vi "Wait on Response.vi"(8 "error in":errorcluster {"code" format="Error %.0f"}, 10 "timeout in ms (-1)":i32=-1, 11 "NATS Subscriber in":refnum<class "NATS Subscription.lvclass">) -> (0 "error out":errorcluster {"code" format="Error %.0f"}, 2 "time out":bool, 3 "nats message":T1)   [LabVIEW 2020, in "NATS Subscription.lvlib" / "NATS Subscription.lvclass"]
doc: "Returns the next subscription response."
uses:
  NATS Subscription.lvclass
  NATS Subscription.lvclass/NATS Subscription.ctl
  <vilib>/NATS/NATS Core/Controls/msg type.ctl
  <vilib>/NATS/NATS Core/NATS Core.lvlib
  <vilib>/NATS/NATS Core/Controls/nats message.ctl
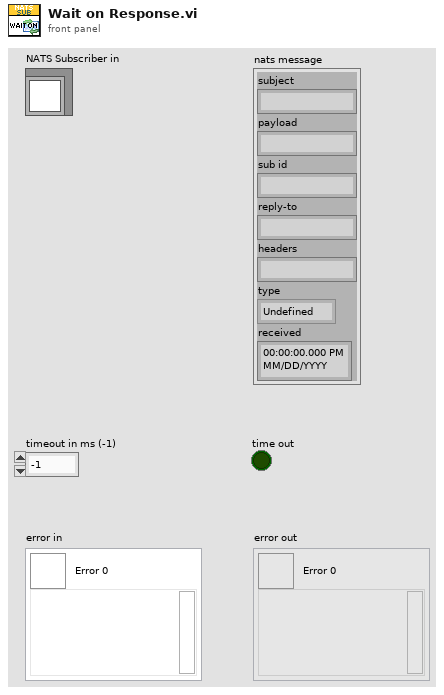
[diagram p1: front panel]
types:
  T1 = typedef "NATS Core.lvlib/nats message.ctl" = cluster{"subject":string, "payload":string, "sub id":string, "reply-to":string, "headers":string, "type":T2, "received":timestamp}
  T2 = typedef "NATS Core.lvlib/msg type.ctl" = enum16{"Undefined", "MSG", "HMSG", "+OK", "PING", "PONG", "-ERR", "INFO"}
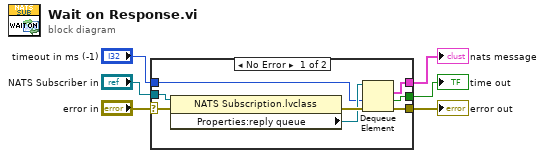
[diagram p0: block diagram]
diagram:
  n1 = case shown="No Error" "error in" {
    selector: "error in" -> [w7 w15]
    tunnel: [w13 w15] -> w6
    tunnel: [w11 _] -> w5
    tunnel: "NATS Subscriber in" -> [w10 _]
    tunnel: "timeout in ms (-1)" -> [w9 _]
    tunnel: [w8 _] -> w2
    frame No Error {
      n2 = property class="NATS Subscription.lvclass"(reference=w10, error in=w7) -> (error out=w14:errorcluster, "Properties:reply queue"=w12:refnum<queue>)  [unwired: 1 out]
      n3 = Dequeue Element(queue=w12, timeout in ms (-1)=w9, error in (no error)=w14) -> (element=w11:T1, timed out?=w8:bool, error out=w13:errorcluster)  [unwired: 1 out]
    }
    frame Error {
    }
  }
  "error out" <- w6
  "nats message" <- w5
  "time out" <- w2
